vi "Sine Wave.vi"() -> ()   [LabVIEW 2020]
uses:
  <vilib>/measure/NI_MABase.lvlib
panel:
  out "X axis Time":dbl
  in  "sampling info":cluster{"Fs":dbl, "#s":dbl}={"Fs"=1000.0, "#s"=1000.0} {"Fs" format="%.2p"}
  out "dt":dbl
  out "Number of Sample":i32
  out "Sine Wave Graph":waveform(dbl)(graph)
  in  "phase":dbl format="%.2p"
  in  "amplitude":dbl(knob)=1.0 scale=0.0..10.0
  in  "frequency":dbl(knob)=10.0 scale=0.0..10.0
  # "in 1 sec there is 1000 samples"
  # "No of samples is #s \nSampling rate is Fs"
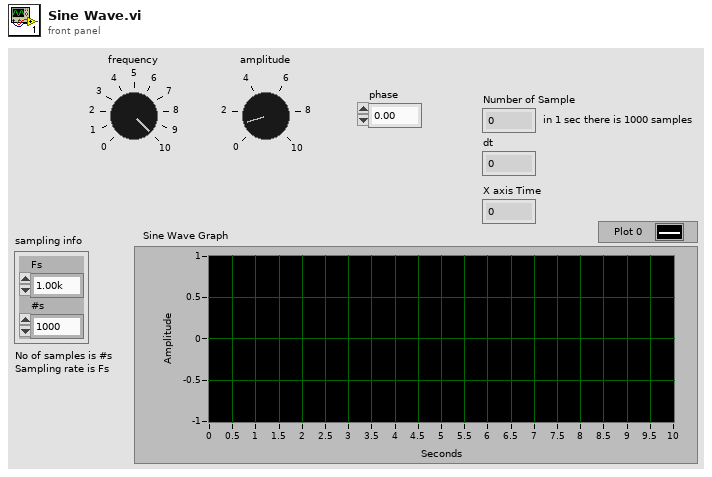
[diagram p1: front panel]
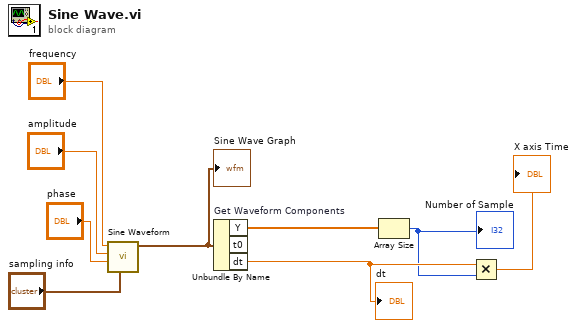
[diagram p0: block diagram]
diagram:
  n1 = call <vilib>:"Sine Waveform.vi"("sampling info"="sampling info", "phase"="phase", "amplitude"="amplitude", "frequency"="frequency") -> ("signal out"=w6:waveform(dbl))  [unwired: 6 in, 1 out]
  "Sine Wave Graph" <- w6
  n2 = Unbundle By Name "Get Waveform Components"(w6) -> ("Y"=w5:dbl[], "dt"=w3:dbl)  [unwired: 1 out]
  "dt" <- w3
  n3 = Array Size(array=w5) -> (size(s)=w2:i32)
  "Number of Sample" <- w2
  n4 = Multiply(x=w3, y=w2) -> (x*y=→"X axis Time":dbl)
